vi "Delete_test_records_by_serial.vi"() -> ()   [LabVIEW 2013]
panel:
  out "error out":errorcluster
  in  "error in":errorcluster
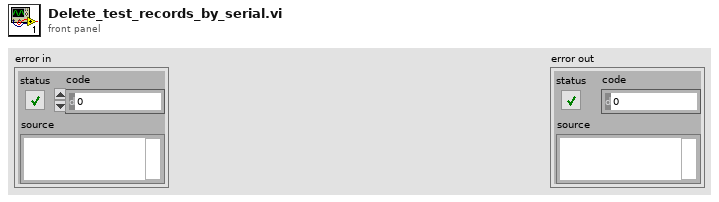
[diagram p1: front panel]
types:
  T1 = enum16{"Query", "Insert", "Select", "Dump Recs", "Get Rec Count", "Get Col Names", "Insert all fields", "Find", "Get last test result", "Get work order qty", "Set work order qty", "Save test report", "Get test report", "Execute query no data", "Select count", "Query and return row 0 col 0"}
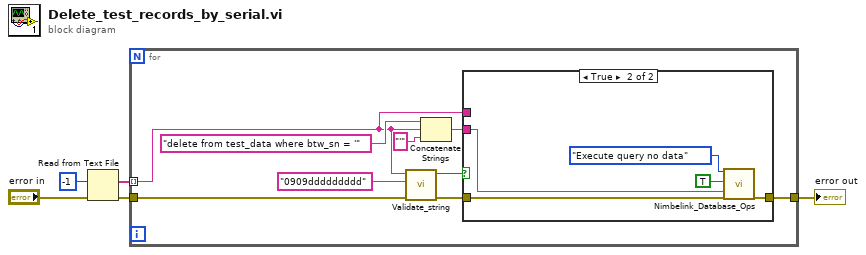
[diagram p0: block diagram]
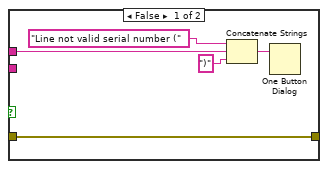
[diagram p2: hidden frame]
diagram:
  n1 = Read from Text File(count=-1, error in="error in") -> (text=w3:string[], error out=w2:errorcluster)  [unwired: 2 in, 2 out]
  n2 = for {
    tunnel: w3 -> [w10] mode=indexing
    tunnel: w2 -> [w12]
    tunnel: [w6] -> w1
    n3 = call "Validate_string.vi"("error in (no error)"=w12, "String data format"="0909ddddddddd", "String"=w10) -> ("error out"=w7:errorcluster, "String Valid"=w11:bool)  [unwired: 7 in]
    n4 = Concatenate Strings("delete from test_data where btw_sn = '" ("string"), w10, "'" ("string")) -> (w8:string)
    n5 = case shown="True" w11 {
      tunnel: w10 -> [w17 _]
      tunnel: w8 -> [_ w23]
      tunnel: w7 -> [w15 w22]
      tunnel: [w15 w21] -> w6
      frame False {
        n6 = Concatenate Strings("Line not valid serial number (" ("string"), w17, ")" ("string")) -> (w19:string)
        n7 = One Button Dialog(message=w19) -> ()  [unwired: 1 in, 1 out]
      }
      frame True {
        n8 = call "Nimbelink_Database_Ops.vi"("Operation"=T1."Execute query no data", "Open SQL session?"=TRUE, "SQL Query"=w23, "Error in (no error)"=w22) -> ("Error out"=w21:errorcluster)  [unwired: 8 in, 7 out]
      }
    }
  }
  "error out" <- w1
